vi "Stack Frame Count (SubVI).vi"(5 "Image Height":u16, 7 "Image Width":u16, 8 "Pixel Valid?":bool) -> (0 "Frame 180?":bool, 3 "Frame 1":bool)   [LabVIEW 2015]
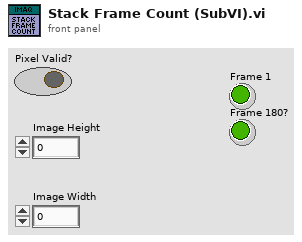
[diagram p1: front panel]
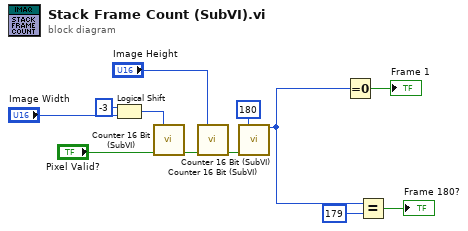
[diagram p0: block diagram]
diagram:
  n1 = Logical Shift(y=i16 -3, x="Image Width") -> (x << y=w7:u16)
  n2 = call "Counter 16 Bit (SubVI).vi"("Max. Count"=w7, "Enable"="Pixel Valid?") -> ("Count End?"=w8:bool)  [unwired: 11 in, 2 out]
  n3 = call "Counter 16 Bit (SubVI).vi"("Max. Count"="Image Height", "Enable"=w8) -> ("Count End?"=w10:bool)  [unwired: 11 in, 2 out]
  n4 = call "Counter 16 Bit (SubVI).vi"("Max. Count"=u16 180, "Enable"=w10) -> ("Count"=w3:u16)  [unwired: 11 in, 2 out]
  n5 = Equal To 0?(x=w3) -> (x = 0?=→"Frame 1":bool)
  n6 = Equal?(x=w3, y=u16 179) -> (x = y?=→"Frame 180?":bool)
